vi "StoppGalvo.vi"(2 "error in":errorcluster, 3 "Galvo-resource in":T2) -> (0 "error out":errorcluster, 1 "Galvo-resource out":T2)   [LabVIEW 2011]
uses:
  SIAM/SIAM-send.ctl
panel:
  out "Stop type":T1(ring)
  out "killed":bool
  out "read 0=succes":string="X\n0\rC\nAV,0,3,-228874\r\nAV,0,4,-228874\r\nAV,0,5,0\r\nAI,0,3,458\r\nAI,0,4,0\r\nAI,0,5,0\r\nAV,80,1,2\r\nAS,80,9,10\r\nAI,1000,3,0\r\nAI,1000,4,2861\r\nAI,1000,5,0\r\nAI,1008,3,-458\r\nAI,1008,4,0\r\nAI,1008,5,0\r\nAV,1080,1,3\r\nAV,1088,1,2\r\nAI,2008,3,0\r\nAI,2008,4,2861\r\nAI,2008,5,0\r\nAI,2016,3,458\r\nAI,2016,4,0\r\nAI,2016,5,0\r\nAV,2088,1,3\r\nAV,2096,1,2\r\nAE,2096,9,0\r\nAV,20240,1,0\r\nAI,20240,3,0\r\nAI,20240,4,0\r\nAI,20240,5,0\r\n"
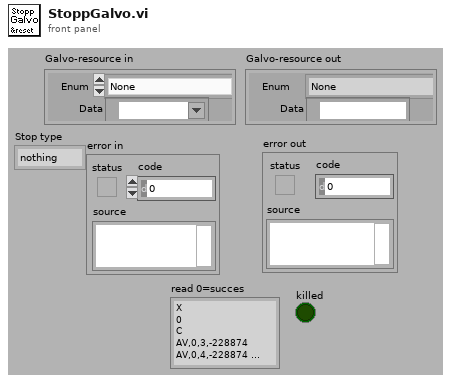
[diagram p1: front panel]
types:
  T1 = enum16{"nothing", "usual", "critical", "emergency"}
  T2 = cluster{"Enum":enum16{"None", "DSP-on serial port", "Analog out", "SIAM-withDSiam"}, "Data":refnum<k21>}
  T3 = enum16{"None", "DSP-on serial port", "Analog out", "SIAM-withDSiam"}
  T4 = typedef "SIAM-send.ctl" = enum16{"validID", "storeID", "enable", "rundirect", "sendlist", "run", "stop", "readRegister", "sendValue", "storeStatus"}
  T5 = enum16{"nothing", "usual", "critical", "emergency"}[]
  T6 = typedef "SIAM_command.ctl" = u32
  T7 = cluster{"Delay 10µs":u32, "command":T6, "P0":i32, "P1":i32, "P2":i32, "P3":i32, "P4":i32, "P5-ticket":i32}[]
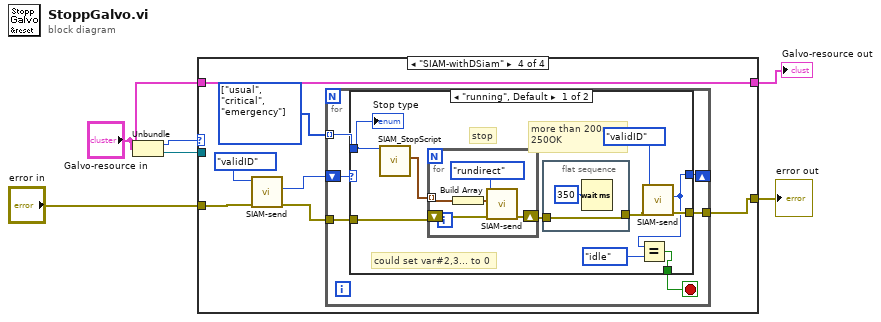
[diagram p0: block diagram]
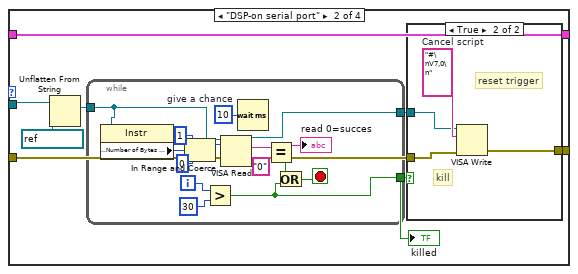
[diagram p3: hidden frame]
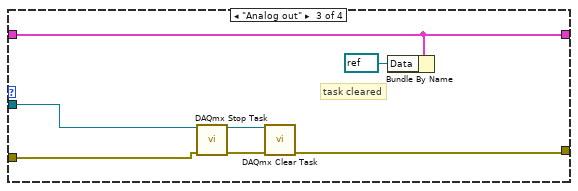
[diagram p5: hidden frame]
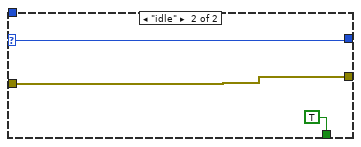
[diagram p6: hidden frame]
diagram:
  n1 = Unbundle("Galvo-resource in") -> ("Enum"=w4:T3, "Data"=w3:refnum<k21>)
  n2 = case shown="\"SIAM-withDSiam\"" w4 {
    tunnel: "error in" -> [w8 w16 w41 w46]
    tunnel: [w8 w15 w36 w49] -> w5
    tunnel: w3 -> [_ w14 w42 _]
    tunnel: "Galvo-resource in" -> [w7 w9 w38 w48]
    tunnel: [w7 w9 w38 w48] -> w1
    frame "None", Default {
    }
    frame "DSP-on serial port" {
      n3 = Unflatten From String(type=refnum<visa-resource-name> "COM1" ("DSP resource name out"), binary string=w14) -> (value=w12:refnum<visa-resource-name>)  [unwired: 1 in, 4 out]
      n4 = while {
        tunnel: w12 -> [w26]
        tunnel: [w33] -> w11
        tunnel: [w27] -> w10
        i -> [w32]
        stop <- w29 stop-if-true
        w34 = u32 10  # give a chance
        n5 = property class="Instr"(reference=w26) -> ("Serial Settings:Number of Bytes at Serial Port"=w25:u32)  [unwired: 1 in, 2 out]
        n6 = In Range and Coerce(upper limit=u32 1, x=w25, lower limit=u32 0) -> (coerced(x)=w24:u32)  [unwired: 1 out]
        n7 = Greater?(x=w32, y=30) -> (0:w27:bool)
        n8 = VISA Read(VISA resource name=w26, byte count=w24) -> (VISA resource name out=w33:refnum<visa-resource-name>, read buffer=w28:string)  [unwired: 1 in, 2 out]
        "read 0=succes" <- w28
        n9 = Wait (ms)(milliseconds to wait=w34) -> ()  [unwired: 1 out]
        n10 = Equal?(x=w28, y="0") -> (x = y?=w30:bool)
        n11 = Or(x=w30, y=w27) -> (x .or. y?=w29:bool)
      }
      "killed" <- w10
      n12 = case shown="True" w10 {
        tunnel: w16 -> [w17 w21]
        tunnel: [w17 w20] -> w15
        tunnel: w11 -> [_ w18]
        frame False {
        }
        frame True {
          w19 = "#\nV7,0\n"  # Cancel script
          # "reset trigger"
          # "kill"
          n13 = VISA Write(VISA resource name=w18, write buffer=w19, error in (no error)=w21) -> (error out=w20:errorcluster)  [unwired: 2 out]
        }
      }
    }
    frame "Analog out" {
      # "task cleared"
      n14 = call <vilib>:"DAQmx Stop Task.vi"("task/channels in"=w42, "error in"=w41) -> ("task out"=w39:refnum<k21>, "error out"=w40:errorcluster)  [unwired: 12 out]
      n15 = call <vilib>:"DAQmx Clear Task.vi"("task in"=w39, "error in"=w40) -> ("error out"=w36:errorcluster)  [unwired: 13 out]
      n16 = Bundle By Name(cluster=w38, "Data"=refnum<k21> refnum) -> ()  [unwired: 1 out]
    }
    frame "SIAM-withDSiam" {
      w43 = T5 [enum."usual", enum."critical", enum."emergency"] items=["nothing", "usual", "critical", "emergency"]
      n17 = call "SIAM-send.vi"("error in (no error)"=w46, "command"=SIAM-send."validID") -> ("error out"=w45:errorcluster, "Status"=w44:enum16{"unknown", "idle", "running", ""})  [unwired: 8 in]
      n18 = for {
        tunnel: [w55] -> w49
        tunnel: w45 -> [w54]
        tunnel: w43 -> [w52] mode=indexing
        shift-right: [w51] -> _
        shift-left: w44 -> [w53]
        stop <- w50 stop-if-true
        n19 = case shown="\"running\", Default" w53 {
          selector: w53 -> [_ w73]
          tunnel: [w64 w75] -> w55
          tunnel: w54 -> [w65 w75]
          tunnel: w52 -> [w59 _]
          tunnel: [w57 w73] -> w51
          tunnel: [w58 TRUE] -> w50
          frame "running", Default {
            # "more than 200ms,\n250OK"
            # "could set var#2,3... to 0"
            # "stop"
            n20 = call "SIAM_StopScript.vi"("Stop type"=w59) -> ("Activate commands (direkt)"=w62:T7)  [unwired: 9 in, 1 out]
            n21 = for {
              tunnel: w62 -> [w69] mode=indexing
              shift-right: [w70] -> w61
              shift-left: w65 -> [w72]
              n22 = Build Array(w69) -> (w68:T7)
              n23 = call "SIAM-send.vi"("error in (no error)"=w72, "Script"=w68, "command"=SIAM-send."rundirect") -> ("error out"=w70:errorcluster)  [unwired: 7 in, 1 out]
            }
            n24 = flat-sequence {
              tunnel: w61 -> [w67]
              tunnel: [w67] -> w60
              frame #0 {
                n25 = Wait (ms)(milliseconds to wait=u32 350) -> ()  [unwired: 1 out]
              }
            }
            n26 = call "SIAM-send.vi"("error in (no error)"=w60, "command"=SIAM-send."validID") -> ("error out"=w64:errorcluster, "Status"=w57:enum16{"unknown", "idle", "running", ""})  [unwired: 8 in]
            n27 = Equal?(x=w57, y=enum16{"unknown", "idle", "running", ""}."idle") -> (x = y?=w58:bool)
            "Stop type" <- w59
          }
          frame "idle" {
          }
        }
      }
    }
  }
  "error out" <- w5
  "Galvo-resource out" <- w1
